vi "FPGA Get Sample Status.vi"(11 "Sample Period (uSec)":u32) -> (0 "error out":errorcluster, 2 "Sample Gated":bool, 3 "Overwrite":bool)   [LabVIEW 2014]
uses:
  <vilib>/rvi/eio/common/nirviEmuClasses.ctl
  <vilib>/rvi/Emulation/niFpgaGetClockAttributes.vi
  <vilib>/rvi/Emulation/niFpgaSctlEmulationGetInTimedLoop.vi
  <vilib>/rvi/Emulation/niFpgaEmulationReportErrorSimple.vi
  FPGA Globals.vi
  <vilib>/rvi/eio/common/nirviEmuTemplateMethod_errors.vi
  <vilib>/rvi/Emulation/niFpgaProcessEmulError.vi
  <vilib>/rvi/Emulation/niFpgaCriticalErrorInLSC.vi
  <vilib>/eio/EIOGrowableMethodNode/genericMethod/EIOGrowableMethodNode.xnode
  <vilib>/rvi/eio/nirviEIOMethodImplementation/nirviEIOMethodImplementation.xnode
  <vilib>/rvi/eio/nirviErrorMerge/nirviErrorMerge.xnode
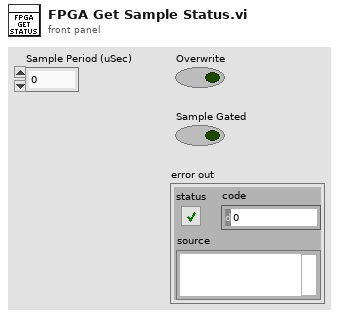
[diagram p1: front panel]
types:
  T1 = typedef "nirviEmuClasses.ctl" = enum16{"IO Read", "IO Write", "Method", "Property Read", "Property Write"}
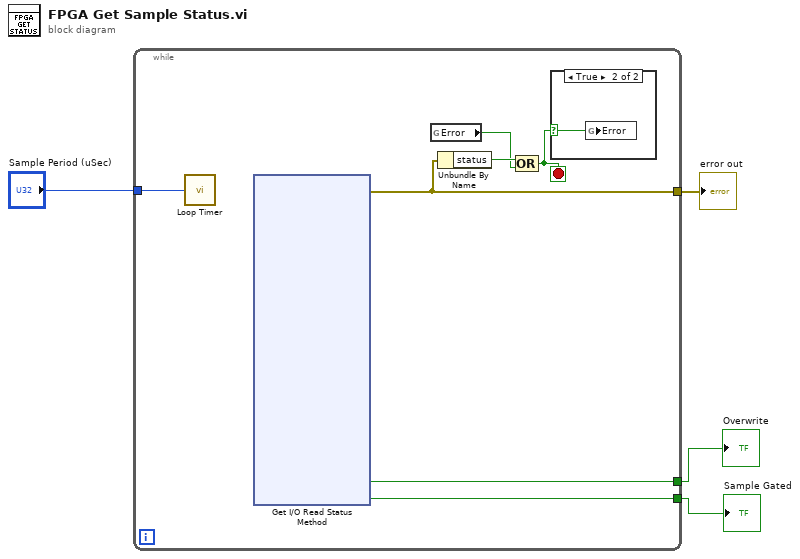
[diagram p0: block diagram]
diagram:
  n1 = while {
    tunnel: [w7] -> w4
    tunnel: "Sample Period (uSec)" -> [w11]
    tunnel: [w5] -> w2
    tunnel: [w6] -> w1
    stop <- w9 stop-if-true
    n2 = call "Loop Timer"("Count(uSec)"=w11) -> ()  [unwired: 1 out]
    n3 = xnode "Get I/O Read Status Method"() -> ("error out"=w7:errorcluster, "Overwrite"=w6:bool, "Sample Gated"=w5:bool)  [unwired: 17 in, 16 out]
    n4 = global read "FPGA Globals.vi" "Error"() -> (w8:bool)
    n5 = Unbundle By Name(w7) -> ("status"=w10:bool)
    n6 = Compound Arithmetic op=OR(w10, w8) -> (w9:bool)
    n7 = case shown="True" w9 {
      selector: w9 -> [_ w576]
      frame False {
      }
      frame True {
        n8 = global write "FPGA Globals.vi" "Error"(w576) -> ()
      }
    }
  }
  "Sample Gated" <- w2
  "Overwrite" <- w1
  "error out" <- w4
